vi "Limit Vector Magnitude.vi"(8 "error in":errorcluster, 9 "Min Magnitude (1)":dbl=1.0, 10 "Max Magnitude (1)":dbl=1.0, 11 "PVector in":refnum<class "PVector.lvclass">) -> (0 "error out":errorcluster, 3 "PVector out":refnum<class "PVector.lvclass">)   [LabVIEW 2016, in "PVector.lvclass"]
doc: "Limits vector magnitude to defined Max and Min thresholds. Is the vector magnitude is within the limit band, the vector is unchanged."
uses:
  PVector.lvclass
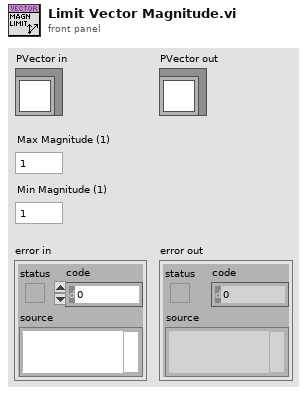
[diagram p1: front panel]
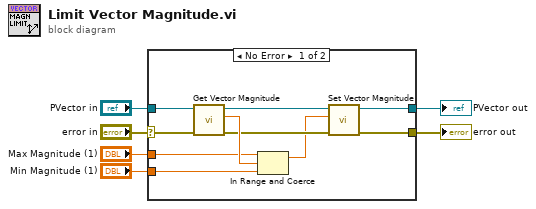
[diagram p0: block diagram]
diagram:
  n1 = case shown="No Error" "error in" {
    selector: "error in" -> [w14 w18]
    tunnel: [w7 w18] -> w5
    tunnel: [w8 w17] -> w3
    tunnel: "PVector in" -> [w16 w17]
    tunnel: "Max Magnitude (1)" -> [w13 _]
    tunnel: "Min Magnitude (1)" -> [w12 _]
    frame No Error {
      n2 = call "Get Vector Magnitude.vi"("error in"=w14, "PVector in"=w16) -> ("error out"=w11:errorcluster, "Mag(V)"=w15:dbl, "PVector out"=w9:refnum<class "PVector.lvclass">)  [unwired: 7 in]
      n3 = In Range and Coerce(upper limit=w13, x=w15, lower limit=w12) -> (coerced(x)=w10:dbl)  [unwired: 1 out]
      n4 = call "Set Vector Magnitude.vi"("error in"=w11, "Manitude"=w10, "PVector in"=w9) -> ("error out"=w7:errorcluster, "PVector out"=w8:refnum<class "PVector.lvclass">)  [unwired: 7 in]
    }
    frame Error {
    }
  }
  "error out" <- w5
  "PVector out" <- w3
